vi "Autosetup.vi"(8 "error in (no error)":errorcluster, 11 "Osciloscopio in":refnum<class "Osciloscopio.lvclass">) -> (0 "error out":errorcluster, 3 "Osciloscopio out":refnum<class "Osciloscopio.lvclass">)   [LabVIEW 2020, in "Oscilloscope.lvlib" / "Osciloscopio.lvclass"]
uses:
  Osciloscopio.lvclass
  Osciloscopio.lvclass/Osciloscopio.ctl
  <instrlib>/Tektronix TDS 200 1000 2000 Series/Tektronix TDS 200 1000 2000 Series.lvlib
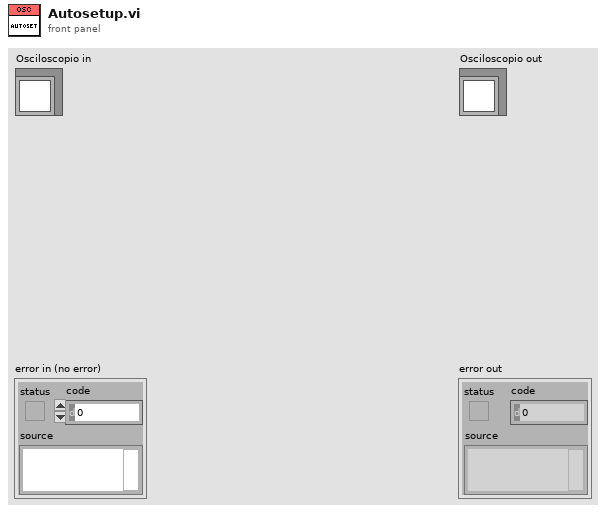
[diagram p1: front panel]
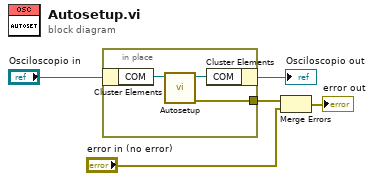
[diagram p0: block diagram]
diagram:
  n1 = in-place {
    in-place-border: [w6] -> w1
    n2 = in-place-cluster #1("Osciloscopio in") -> ("COM"=w8:refnum<visa-resource-name>)
    n3 = call <instrlib>:"Autosetup.vi"("VISA resource name"=w8) -> ("error out"=w6:errorcluster, "VISA resource name out"=w7:refnum<visa-resource-name>)  [unwired: 9 in]
    n4 = in-place-cluster #1("COM"=w7) -> (→"Osciloscopio out":refnum<class "Osciloscopio.lvclass">)
  }
  n5 = Merge Errors(w1, "error in (no error)") -> (→"error out":errorcluster)
